vi "xps_get_positioner_names.vi"(8 "error in (no error)":errorcluster, 11 "newport_xps in":refnum<class "newport_xps.lvclass">) -> (0 "error out":errorcluster, 2 "Positioners":string[](array[string]), 3 "newport_xps out":refnum<class "newport_xps.lvclass">)   [LabVIEW 2015, in "newport_xps.lvclass"]
uses:
  newport_xps.lvclass
  newport_xps.lvclass/newport_xps.ctl
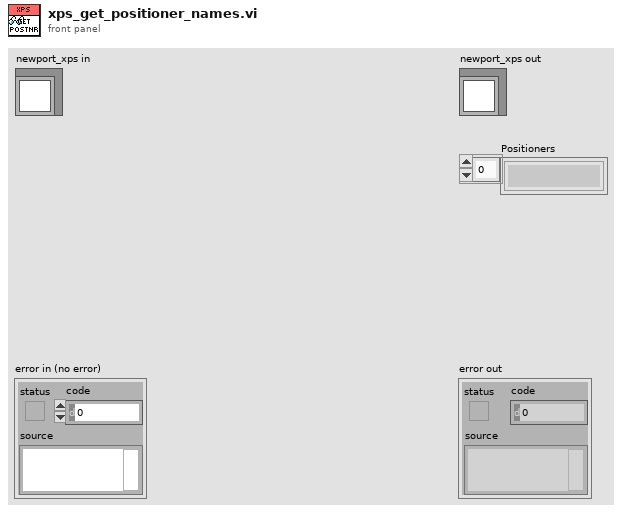
[diagram p1: front panel]
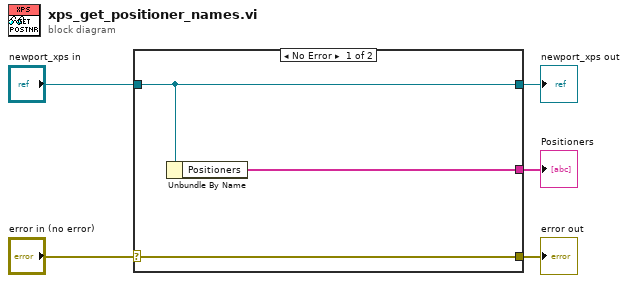
[diagram p0: block diagram]
diagram:
  n1 = case shown="No Error" "error in (no error)" {
    selector: "error in (no error)" -> [w8 w9]
    tunnel: [w8 w9] -> w4
    tunnel: [w7 w10] -> w2
    tunnel: "newport_xps in" -> [w7 w10]
    tunnel: [w6 _] -> w1
    frame No Error {
      n2 = Unbundle By Name(w7) -> ("Positioners"=w6:string[])
    }
    frame Error {
    }
  }
  "error out" <- w4
  "newport_xps out" <- w2
  "Positioners" <- w1
